vi "XML Get attribute value.vi"(8 "error in (no error)":errorcluster, 10 "Attribute name":string, 11 "Tag node":refnum<k20>) -> (0 "error out":errorcluster, 2 "Attribute value":string, 3 "Tag node out":refnum<k20>)   [LabVIEW 2014, in "COSYLib.lvlib"]
uses:
  COSYLib.lvlib
  <vilib>/xml/Close Reference(Node).vi
  <vilib>/xml/Close Reference(NNMap).vi
  <resource>/objmgr/DOMUserDefRef.rc
  <vilib>/xml/NI_XML.lvlib
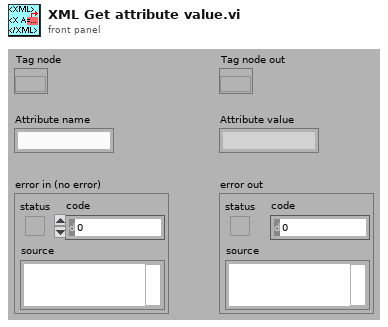
[diagram p1: front panel]
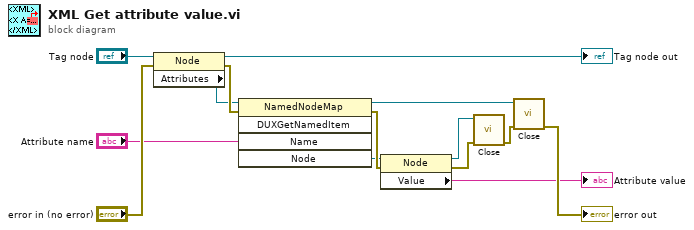
[diagram p0: block diagram]
diagram:
  n1 = property class="Node"(reference="Tag node", error in="error in (no error)") -> (reference out=→"Tag node out":refnum<k20>, error out=w11:errorcluster, "Attributes"=w9:refnum<k20>)
  n2 = invoke class="NamedNodeMap" method="DUXGetNamedItem"(reference=w9, error in=w11, "Name"="Attribute name") -> (reference out=w5:refnum<k20>, error out=w10:errorcluster, "Node"=w7:refnum<k20>)  [unwired: 2 in, 2 out]
  n3 = property class="Node"(reference=w7, error in=w10) -> (reference out=w4:refnum<k20>, error out=w2:errorcluster, "Value"=→"Attribute value":string)
  n4 = call-poly <vilib>:"Close.vi"("error in (no error)"=w2, "node"=w4) -> ("error out"=w3:errorcluster)  [unwired: 7 in]
  n5 = call-poly <vilib>:"Close.vi"("error in (no error)"=w3, "named node map"=w5) -> ("error out"=→"error out":errorcluster)  [unwired: 7 in]
